vi "Generate Event.vi"(8 "error in (no error)":errorcluster, 10 "opcode (text)":T1=1 items=["Cont. Frame"=0, "Text"=1, "Binary"=2, "Close Frame"=8, "Ping"=9, "Pong"=10], 11 "device data model in":refnum<class "WebSocket Data Model.lvclass">) -> (0 "error out":errorcluster, 3 "device data model out":refnum<class "WebSocket Data Model.lvclass">)   [LabVIEW 2021, in "WebSockets.lvlib" / "WebSocket Data Model.lvclass"]
doc: "This VI initializes the device data model."
uses:
  WebSocket Data Model.lvclass
  WebSocket/Opcodes.ctl
  WebSocket Data Model.lvclass/WebSocket Data Model.ctl
  WebSocket/WebSocket.lvclass
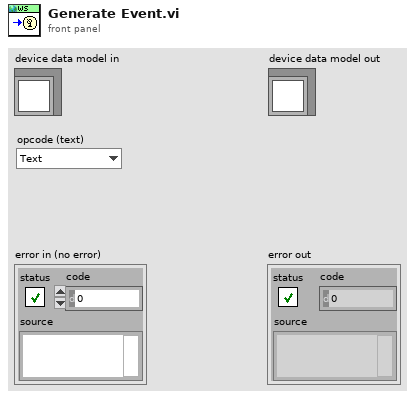
[diagram p1: front panel]
types:
  T1 = typedef "WebSockets.lvlib/WebSocket.lvclass/Opcodes.ctl" = u8
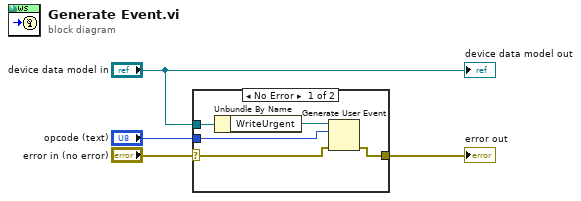
[diagram p0: block diagram]
diagram:
  n1 = case shown="No Error" "error in (no error)" {
    selector: "error in (no error)" -> [w6 w10]
    tunnel: "device data model in" -> [w9 _]
    tunnel: [w5 w10] -> w3
    tunnel: "opcode (text)" -> [w7 _]
    frame No Error {
      n2 = Unbundle By Name(w9) -> ("WriteUrgent"=w8:refnum<user-event>)
      n3 = Generate User Event(user event=w8, event data cluster=w7, error in=w6) -> (error out=w5:errorcluster)  [unwired: 1 in, 1 out]
    }
    frame Error {
    }
  }
  "error out" <- w3
  "device data model out" <- "device data model in"
